vi "Turret_Desired_Position_Control.vi"(6 "Found Target?":bool, 7 "Current Position":dbl, 8 "Reset Turret?":bool, 9 "Aim with Camera?":bool, 10 "Camera Desired Position Change":dbl, 11 "User Position Change Command":dbl) -> (3 "Desired Position":dbl)   [LabVIEW 2012]
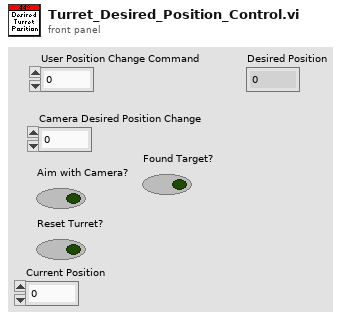
[diagram p1: front panel]
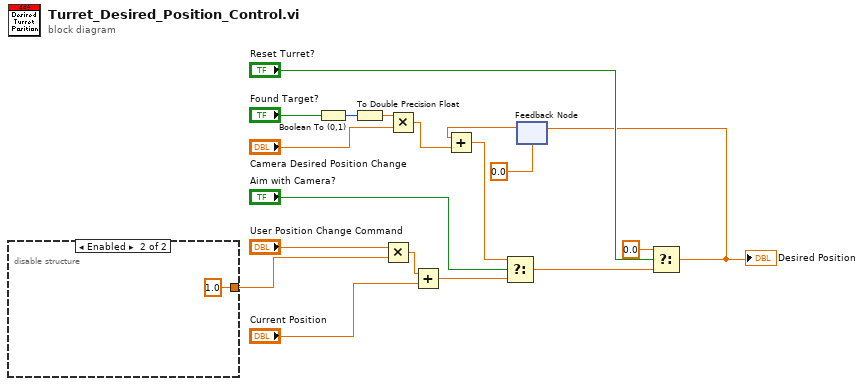
[diagram p0: block diagram]
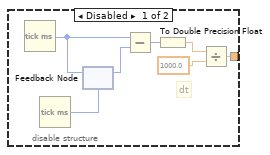
[diagram p2: hidden frame]
diagram:
  n1 = disable-structure shown="Enabled" {
    disable-tunnel: [w25 1.0] -> w18
    frame Disabled {
      # "dt"
      n2 = Tick Count (ms)() -> (millisecond timer value=w21:u32)
      n3 = Tick Count (ms)() -> (millisecond timer value=w19:u32)
      n4 = feedback #1(w19) -> (w20:u32)
      n5 = feedback-in #1(w21) -> ()
      n6 = Subtract(x=w21, y=w20) -> (x-y=w22:u32)
      n7 = To Double Precision Float(number=w22) -> (double precision float=w23:dbl)
      n8 = Divide(x=w23, y=1000.0) -> (x/y=w25:dbl)
    }
    frame Enabled {
    }
  }
  n9 = Boolean To (0,1)(Boolean="Found Target?") -> (0, 1=w4:i16)
  n10 = To Double Precision Float(number=w4) -> (double precision float=w2:dbl)
  n11 = Multiply(x="User Position Change Command", y=w18) -> (x*y=w10:dbl)
  n12 = Multiply(x=w2, y="Camera Desired Position Change") -> (x*y=w1:dbl)
  n13 = Add(x=w10, y="Current Position") -> (x+y=w12:dbl)
  n14 = feedback #2(0.0 ("Camera Desired Position")) -> (w6:dbl)
  n15 = Add(x=w6, y=w1) -> (x+y=w8:dbl)
  n16 = Select(t=w8, s="Aim with Camera?", f=w12) -> (s? t:f=w7:dbl)
  n17 = Select(t=0.0, s="Reset Turret?", f=w7) -> (s? t:f=w13:dbl)
  "Desired Position" <- w13
  n18 = feedback-in #2(w13) -> ()
